vi "LaserStartUpSequence.vi"(8 "error in (no error)":errorcluster) -> (0 "error out":errorcluster)   [LabVIEW 2013]
uses:
  Variables/405Pico.vi
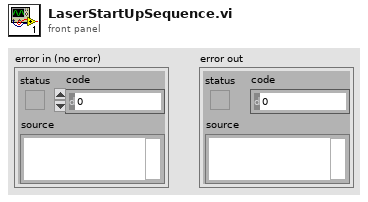
[diagram p1: front panel]
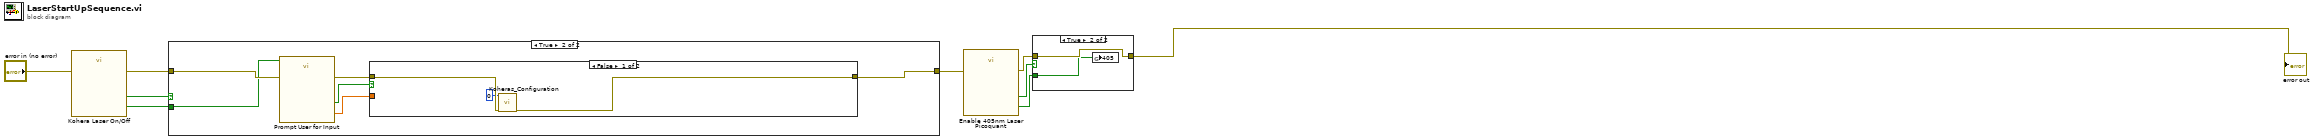
[diagram p0: block diagram]
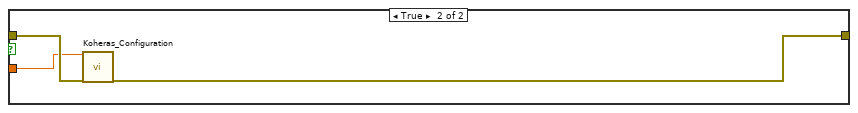
[diagram p3: hidden frame]
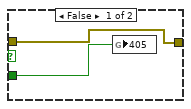
[diagram p4: hidden frame]
diagram:
  n1 = call "Kohera Laser On/Off"("error in (no error)"="error in (no error)") -> ("Koheras Laser On/Off"=w9:bool, "OK"=w8:bool, "error out"=w7:errorcluster)  [unwired: 16 in]
  n2 = case shown="True" w8 {
    tunnel: [w10 w13] -> w2
    tunnel: w7 -> [w10 w12]
    tunnel: w9 -> [_ w11]
    frame False {
    }
    frame True {
      n3 = call "Prompt User for Input"("Enable"=w11, "error in (no error)"=w12) -> ("Laser Power"=w15:dbl, "OK"=w14:bool, "error out"=w16:errorcluster)  [unwired: 15 in]
      n4 = case shown="False" w14 {
        tunnel: [w18 w22] -> w13
        tunnel: w16 -> [w19 w21]
        tunnel: w15 -> [_ w20]
        frame False {
          n5 = call "Koheras_Configuration.vi"("laserPower"=0, "error in"=w19) -> ("out"=w18:errorcluster)  [unwired: 17 in]
        }
        frame True {
          n6 = call "Koheras_Configuration.vi"("laserPower"=w20, "error in"=w21) -> ("out"=w22:errorcluster)  [unwired: 17 in]
        }
      }
    }
  }
  n7 = call "Enable 405nm Laser Picoquant"("error in (no error)"=w2) -> ("On/Off"=w5:bool, "OK"=w4:bool, "error out"=w3:errorcluster)  [unwired: 16 in]
  n8 = case shown="True" w4 {
    tunnel: [w24 w26] -> w1
    tunnel: w3 -> [w24 w26]
    tunnel: w5 -> [w23 w25]
    frame False {
      n9 = global write "405Pico.vi" "405"(w23) -> ()
    }
    frame True {
      n10 = global write "405Pico.vi" "405"(w25) -> ()
    }
  }
  "error out" <- w1
